vi "KnifeEdge_Intensity_simulation.vi"(5 "w_0":dbl=0.002, 7 "Z_0":dbl=0.1, 9 "Z":dbl=1.0, 10 "X":dbl) -> (2 "E":dbl)   [LabVIEW 2012]
doc: "This template is the starting point for creating a model function to be passed to the Nonlinear Curve Fit.vi."
uses:
  <vilib>/gmath/NI_Gmath.lvlib
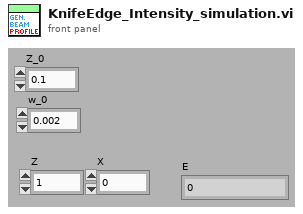
[diagram p1: front panel]
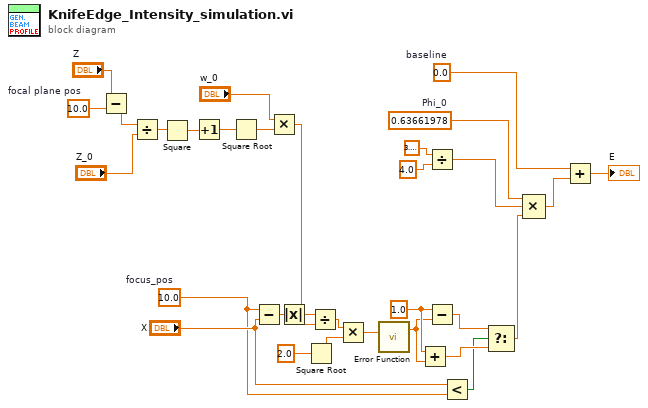
[diagram p0: block diagram]
diagram:
  w1 = 10.0  # focal plane pos
  w12 = 10.0  # focus_pos
  w6 = 0.0  # baseline
  w7 = 0.63661978  # Phi_0
  w19 = 1.0 ("x")
  n1 = Subtract(x="Z", y=w1) -> (x-y=w2:dbl)
  n2 = Divide(x=w2, y="Z_0") -> (x/y=w26:dbl)
  n3 = Square(x=w26) -> (x^2=w3:dbl)
  n4 = Increment(x=w3) -> (x+1=w25:dbl)
  n5 = Square Root(x=w25) -> (sqrt(x)=w11:dbl)
  n6 = Subtract(x=w12, y="X") -> (x-y=w23:dbl)
  n7 = Multiply(x="w_0", y=w11) -> (x*y=w9:dbl)
  n8 = Absolute Value(x=w23) -> (abs(x)=w22:dbl)
  n9 = Square Root(x=2.0) -> (sqrt(x)=w30:dbl)
  n10 = Divide(x=w22, y=w9) -> (x/y=w21:dbl)
  n11 = Multiply(x=w21, y=w30) -> (x*y=w20:dbl)
  n12 = call <vilib>:"Error Function.vi"("x"=w20) -> ("erf(x)"=w18:dbl)  [unwired: 2 in]
  n13 = Add(x=w19, y=w18) -> (x+y=w16:dbl)
  n14 = Divide(x=3.141592653589793, y=4.0) -> (x/y=w27:dbl)
  n15 = Subtract(x=w19, y=w18) -> (x-y=w17:dbl)
  n16 = Less?(x="X", y=w12) -> (x < y?=w15:bool)
  n17 = Select(t=w17, s=w15, f=w16) -> (s? t:f=w14:dbl)
  n18 = Compound Arithmetic op=MULTIPLY(w7, w27, w14) -> (w24:dbl)
  n19 = Add(x=w6, y=w24) -> (x+y=→"E":dbl)
